vi "MTest.vi"() -> ()   [LabVIEW 2020]
uses:
  Controlword_transition.ctl
  Statusword_status.ctl
  ElementDTD.lvlib
panel:
  in  "Outputs-profile_velocity 2":u32
  in  "Outputs-profile_velocity":u32
  out "Mode_of_operation 2":T1(ring)
  out "Statusword_out 2":bool[](array[boolean])
  in  "halt 2":u16
  in  "Mode_out 2":i8(ring)=1 items=["Profile_Pos"=1, "Profile_Vel"=3, "Torque_Prof"=4, "Homing"=6, "Inter_Pos"=7]
  in  "reset 2":u16
  out "Outputs-mode_of_operation 2":i8
  in  "transition_out 2":T2=3 items=["Disable_Voltage"=0, "Unknown"=3, "Quick_Stop"=2, "Shutdown"=6, "Enable_Operation"=15]
  out "Inputs-statusword 2":u16 format="%b"
  out "controlword 2":u16 format="%b"
  in  "Outputs-target_position 2":i32
  out "Status 2":T3
  out "Inputs-position_actual_value 2":dbl
  in  "new_set_point 2":bool
  out "Inputs-velocity_actual_value 2":i32
  out "Inputs-velocity_actual_value":i32
  in  "new_set_point":bool
  out "Inputs-position_actual_value":dbl
  out "Status":T3
  in  "Outputs-target_position":i32
  out "controlword":u16 format="%b"
  out "Inputs-statusword":u16 format="%b"
  in  "transition_out":T2=3 items=["Disable_Voltage"=0, "Unknown"=3, "Quick_Stop"=2, "Shutdown"=6, "Enable_Operation"=15]
  out "Outputs-mode_of_operation":i8
  in  "reset":u16
  in  "Mode_out":i8(ring)=1 items=["Profile_Pos"=1, "Profile_Vel"=3, "Torque_Prof"=4, "Homing"=6, "Inter_Pos"=7]
  in  "halt":u16
  out "Statusword_out":bool[](array[boolean])
  out "Mode_of_operation":T1(ring)
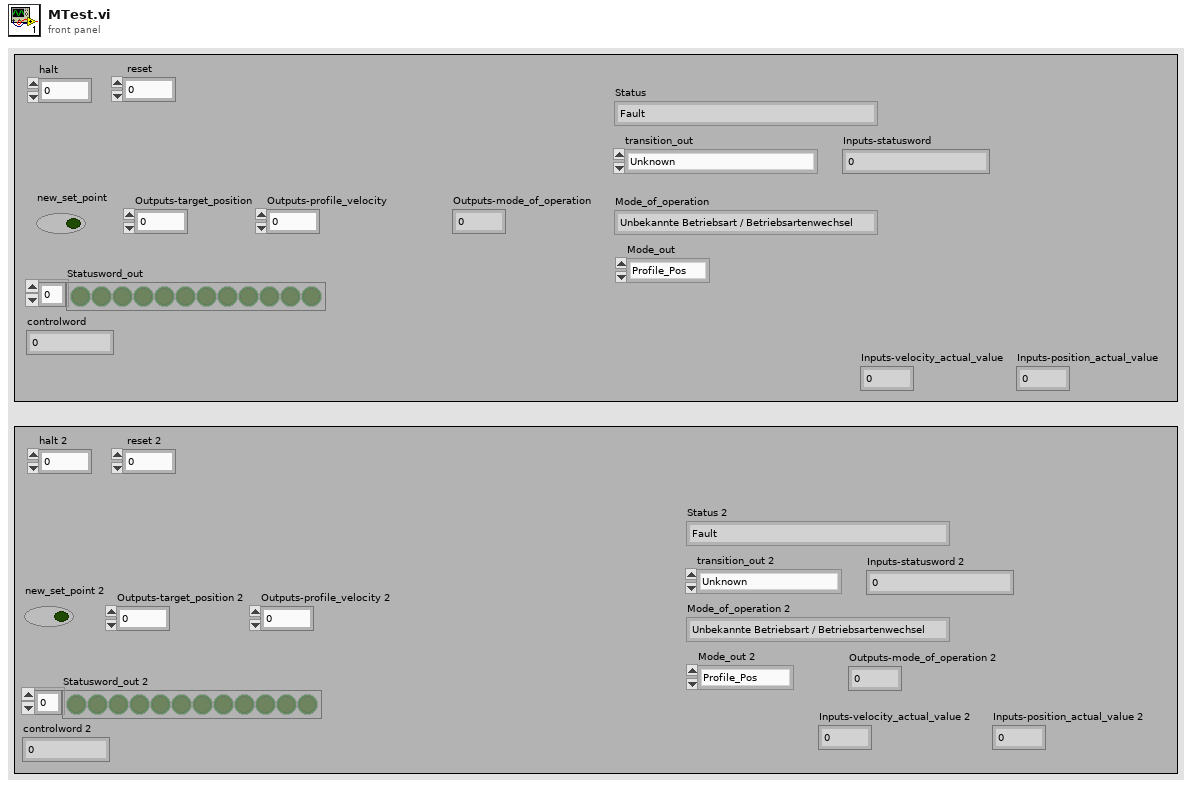
[diagram p1: front panel]
types:
  T1 = enum16{"Unbekannte Betriebsart / Betriebsartenwechsel", "User_position_mode", "User_velocity_mode", "User_torque_mode", "Profile_position_mode", "Profile_velocity_mode", "Torque_profile_mode", "Homing_Mode", "Interpolated_position_mode"}
  T2 = typedef "ElementDTD.lvlib/Controlword_transition.ctl" = u16
  T3 = typedef "ElementDTD.lvlib/Statusword_status.ctl" = enum16{"Fault", "NOT_READY_TO_SWITCH_ON", "SWITCH_ON_DISABLED", "READY_TO_SWITCH_ON", "SWITCHED_ON", "OPERATION_ENABLE", "QUICK_STOP_ACTIVE"}
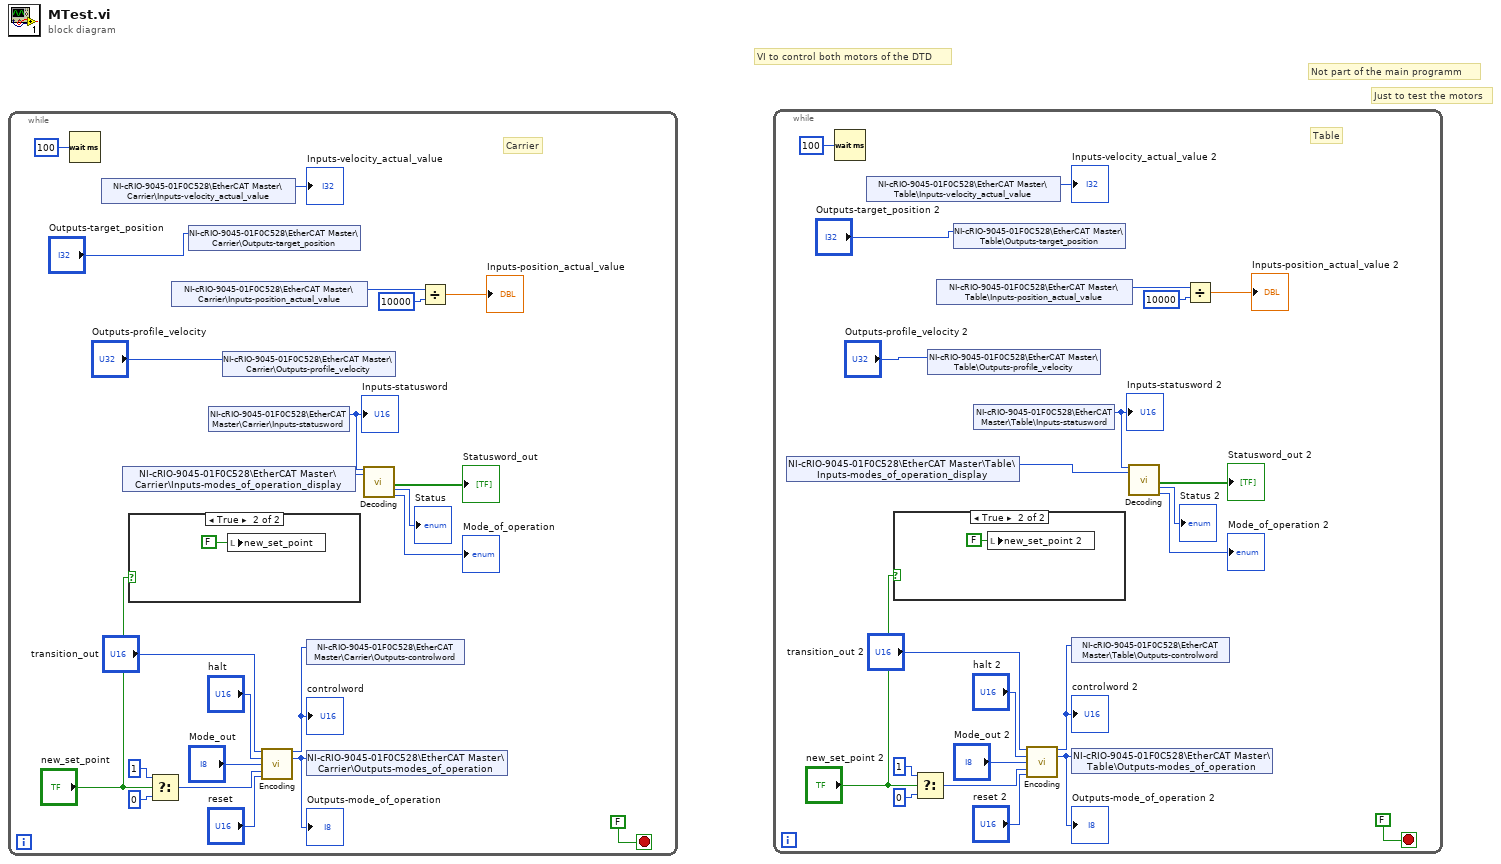
[diagram p0: block diagram]
diagram:
  # "Just to test the motors"
  # "Not part of the main programm"
  # "VI to control both motors of the DTD"
  n1 = while {
    stop <- FALSE stop-if-true
    # "Carrier"
    n2 = Wait (ms)(milliseconds to wait=u32 100) -> ()  [unwired: 1 out]
    n3 = shared-variable "NI-cRIO-9045-01F0C528\\EtherCAT Master\\Carrier\\Inputs-velocity_actual_value"() -> (→"Inputs-velocity_actual_value":i32)  [unwired: 1 in, 1 out]
    n4 = shared-variable "NI-cRIO-9045-01F0C528\\EtherCAT Master\\Carrier\\Inputs-modes_of_operation_display"() -> (w3:i8)  [unwired: 1 in, 1 out]
    n5 = case shown="True" "new_set_point" {
      frame False {
      }
      frame True {
        n6 = local write "new_set_point"(FALSE ("new_set_point")) -> ()
      }
    }
    n7 = Select(t=u16 1 ("new_set_point"), s="new_set_point", f=u16 0 ("new_set_point")) -> (s? t:f=w11:u16)
    n8 = shared-variable "NI-cRIO-9045-01F0C528\\EtherCAT Master\\Carrier\\Inputs-position_actual_value"() -> (w4:i32)  [unwired: 1 in, 1 out]
    n9 = shared-variable "NI-cRIO-9045-01F0C528\\EtherCAT Master\\Carrier\\Outputs-target_position"("Outputs-target_position") -> ()  [unwired: 1 in, 1 out]
    n10 = shared-variable "NI-cRIO-9045-01F0C528\\EtherCAT Master\\Carrier\\Inputs-statusword"() -> (w5:u16)  [unwired: 1 in, 1 out]
    "Inputs-statusword" <- w5
    n11 = shared-variable "NI-cRIO-9045-01F0C528\\EtherCAT Master\\Carrier\\Outputs-profile_velocity"("Outputs-profile_velocity") -> ()  [unwired: 1 in, 1 out]
    n12 = call "Encoding.vi"("transition_out"="transition_out", "halt"="halt", "Mode_out"="Mode_out", "new_set_point"=w11, "reset"="reset") -> ("controlword"=w8:u16, "Outputs-mode_of_operation"=w7:i8)  [unwired: 9 in]
    "Outputs-mode_of_operation" <- w7
    "controlword" <- w8
    n13 = shared-variable "NI-cRIO-9045-01F0C528\\EtherCAT Master\\Carrier\\Outputs-controlword"(w8) -> ()  [unwired: 1 in, 1 out]
    n14 = shared-variable "NI-cRIO-9045-01F0C528\\EtherCAT Master\\Carrier\\Outputs-modes_of_operation"(w7) -> ()  [unwired: 1 in, 1 out]
    n15 = call "Decoding.vi"("Inputs-statusword"=w5, "Input-modes_of_operation_display"=w3) -> ("Statusword_out"=→"Statusword_out":bool[], "Status"=→"Status":T3, "Mode_of_operation"=→"Mode_of_operation":T1)  [unwired: 15 in]
    n16 = Divide(x=w4, y=10000) -> (x/y=→"Inputs-position_actual_value":dbl)
  }
  n17 = while {
    stop <- FALSE stop-if-true
    # "Table"
    n18 = shared-variable "NI-cRIO-9045-01F0C528\\EtherCAT Master\\Table\\Inputs-modes_of_operation_display"() -> (w27:i8)  [unwired: 1 in, 1 out]
    n19 = Wait (ms)(milliseconds to wait=u32 100) -> ()  [unwired: 1 out]
    n20 = shared-variable "NI-cRIO-9045-01F0C528\\EtherCAT Master\\Table\\Inputs-velocity_actual_value"() -> (→"Inputs-velocity_actual_value 2":i32)  [unwired: 1 in, 1 out]
    n21 = case shown="True" "new_set_point 2" {
      frame False {
      }
      frame True {
        n22 = local write "new_set_point 2"(FALSE ("new_set_point")) -> ()
      }
    }
    n23 = Select(t=u16 1 ("new_set_point"), s="new_set_point 2", f=u16 0 ("new_set_point")) -> (s? t:f=w35:u16)
    n24 = shared-variable "NI-cRIO-9045-01F0C528\\EtherCAT Master\\Table\\Outputs-profile_velocity"("Outputs-profile_velocity 2") -> ()  [unwired: 1 in, 1 out]
    n25 = shared-variable "NI-cRIO-9045-01F0C528\\EtherCAT Master\\Table\\Inputs-position_actual_value"() -> (w28:i32)  [unwired: 1 in, 1 out]
    n26 = shared-variable "NI-cRIO-9045-01F0C528\\EtherCAT Master\\Table\\Outputs-target_position"("Outputs-target_position 2") -> ()  [unwired: 1 in, 1 out]
    n27 = shared-variable "NI-cRIO-9045-01F0C528\\EtherCAT Master\\Table\\Inputs-statusword"() -> (w29:u16)  [unwired: 1 in, 1 out]
    "Inputs-statusword 2" <- w29
    n28 = call "Encoding.vi"("transition_out"="transition_out 2", "halt"="halt 2", "Mode_out"="Mode_out 2", "new_set_point"=w35, "reset"="reset 2") -> ("controlword"=w32:u16, "Outputs-mode_of_operation"=w31:i8)  [unwired: 9 in]
    "Outputs-mode_of_operation 2" <- w31
    "controlword 2" <- w32
    n29 = shared-variable "NI-cRIO-9045-01F0C528\\EtherCAT Master\\Table\\Outputs-controlword"(w32) -> ()  [unwired: 1 in, 1 out]
    n30 = shared-variable "NI-cRIO-9045-01F0C528\\EtherCAT Master\\Table\\Outputs-modes_of_operation"(w31) -> ()  [unwired: 1 in, 1 out]
    n31 = call "Decoding.vi"("Inputs-statusword"=w29, "Input-modes_of_operation_display"=w27) -> ("Statusword_out"=→"Statusword_out 2":bool[], "Status"=→"Status 2":T3, "Mode_of_operation"=→"Mode_of_operation 2":T1)  [unwired: 15 in]
    n32 = Divide(x=w28, y=10000) -> (x/y=→"Inputs-position_actual_value 2":dbl)
  }
